vi "MPExxx_get_stat_ques.vi"(0 "VISA session":refnum<visa-resource-name>, 1 "error in (no error)":errorcluster) -> (2 "dup VISA session":refnum<visa-resource-name>, 3 "Questionable Status Register":string, 4 "error out":errorcluster)   [LabVIEW 2012]
doc: "This query returns the value of the Questionable Register. The Questionable Register is a read-only register that holds the real-time (un-latched) condition of the questionable status of the power supply.\n\nBIT DESCRIPTION\n0 - Over Voltage Tripped\n1 - Over Current Tripped\n2 - Phase Balance Protection Tripped\n3 - Program Line Protection Tripped\n4 - Over Temperature Protection Tripped\n5 - Fuse Protection Tripped\n6 - Not used\n7 - Alarm Protection Tripped \n8 - Interlock Alarm\n9 - Remote\n10-15 Not used"
panel:
  # "MAGNA-POWER"
  # "Electronics"
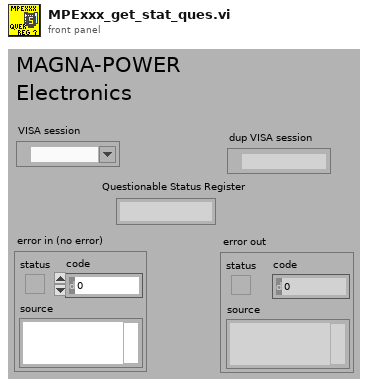
[diagram p1: front panel]
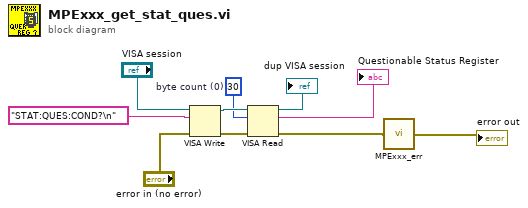
[diagram p0: block diagram]
diagram:
  w8 = u32 30  # byte count (0)
  n1 = VISA Write(VISA resource name="VISA session", write buffer="STAT:QUES:COND?\n", error in (no error)="error in (no error)") -> (VISA resource name out=w9:refnum<visa-resource-name>, error out=w7:errorcluster)  [unwired: 1 out]
  n2 = VISA Read(VISA resource name=w9, byte count=w8, error in (no error)=w7) -> (VISA resource name out=→"dup VISA session":refnum<visa-resource-name>, read buffer=→"Questionable Status Register":string, error out=w2:errorcluster)  [unwired: 1 out]
  n3 = call "MPExxx_err.vi"("error in (no error)"=w2) -> ("error out"=→"error out":errorcluster)
